vi "Streaming to Asset Example.vi"() -> ()   [LabVIEW 2024]
doc: "Streams multiple channels to a Run."
uses:
  Sift API/Sift Client.lvclass
  Generate Sift Protos/SiftProxy_client/RPC Messages/sift_proxy_v1_ChannelDataType.ctl
  Sift Client.lvlib
  Generate Sift Protos/SiftProxy_client/SiftProxy_client.lvlib
panel:
  out "Running":bool
  out "Flush Error":errorcluster
  in  "Test Channel 2":dbl(slide) scale=0.0..10.0
  in  "Stop":bool
  in  "Test Channel 1":dbl(slide) scale=0.0..10.0
  in  "Test Channel 3":bool
  out "Error":errorcluster
  in  "Organization ID":string
  in  "API Key":string
  in  "API URL":string
  # "Sift Streaming Example"
  # "Instructions\n\n1. Fill in the API URL, API Key, and Organization ID. Visit this URL for more information on authentication\n    https://docs.siftstack.com/docs/api/authentication\n\n\n2. Start the VI\n\n3. Navigate to the Assets page and open the \"LabVIEW-Example\" asset.\n\n4. You should see the test test channels in the run.\n\n5. Click on the Live button and manually adjust the Controls to see the telemetry update.\n\n6. Click Stop to stop the VI."
  # "This example streams data live from LabVIEW.\n\nFill in the information below then open the corresponding Run in Sift\nto see data streaming in Live.\n\nNote: Remembver to hit the \"Live\" button after opening the run."
  # "Adjust these values while streaming"
  # "Hit this to stop the example."
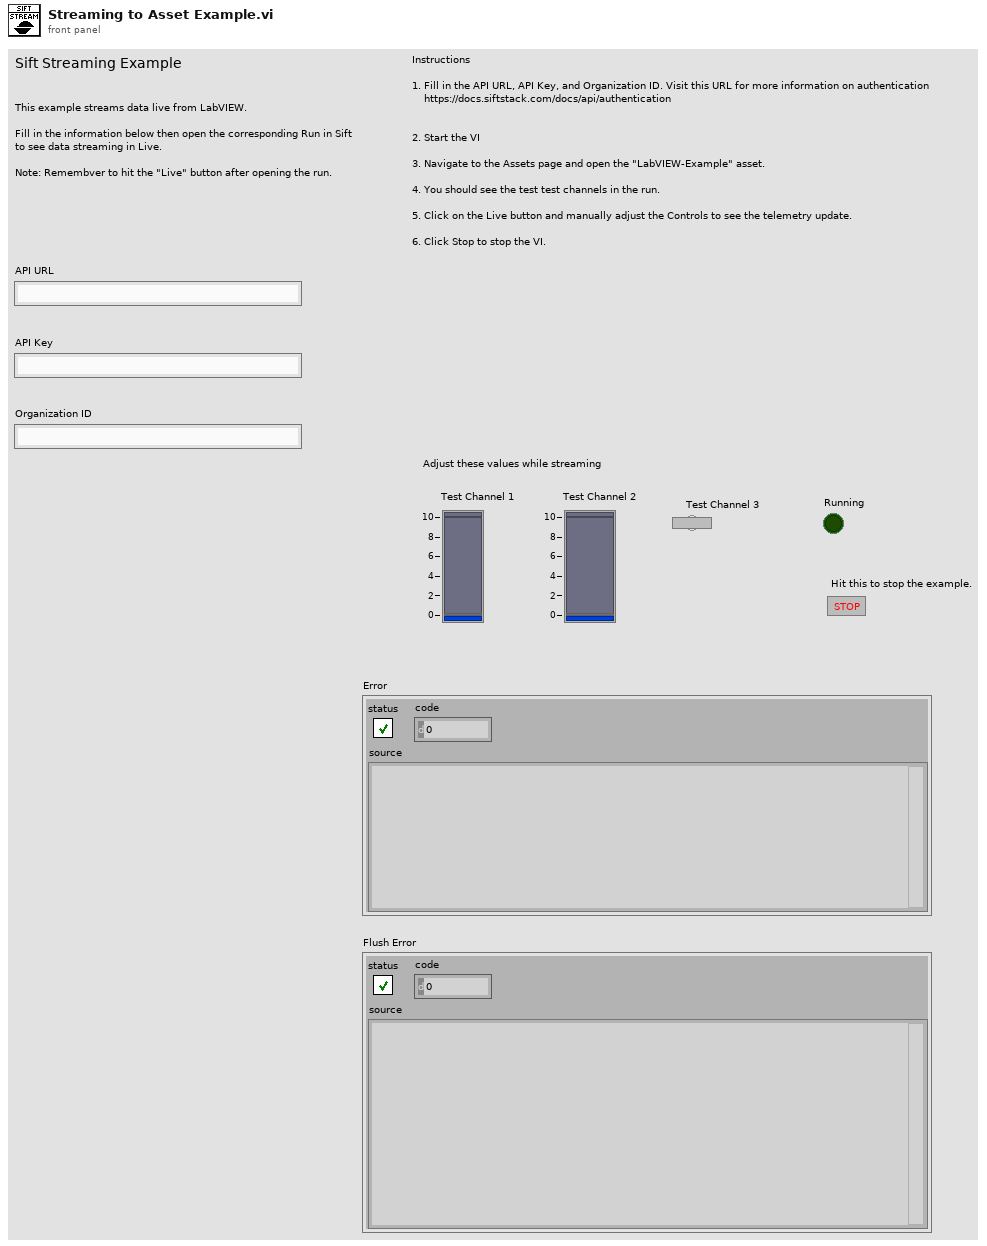
[diagram p1: front panel]
types:
  T1 = typedef "SiftProxy_client.lvlib/sift_proxy_v1_ChannelDataType.ctl" = enum32{"CHANNEL_DATA_TYPE_UNSPECIFIED", "CHANNEL_DATA_TYPE_DOUBLE", "CHANNEL_DATA_TYPE_STRING", "CHANNEL_DATA_TYPE_ENUM", "CHANNEL_DATA_TYPE_BIT_FIELD", "CHANNEL_DATA_TYPE_BOOL", "CHANNEL_DATA_TYPE_FLOAT", "CHANNEL_DATA_TYPE_INT_32", "CHANNEL_DATA_TYPE_UINT_32", "CHANNEL_DATA_TYPE_INT_64", "CHANNEL_DATA_TYPE_UINT_64"}
  T2 = typedef "SiftProxy_client.lvlib/google_protobuf_Timestamp.ctl" = cluster{"seconds":i64, "nanos":i32}
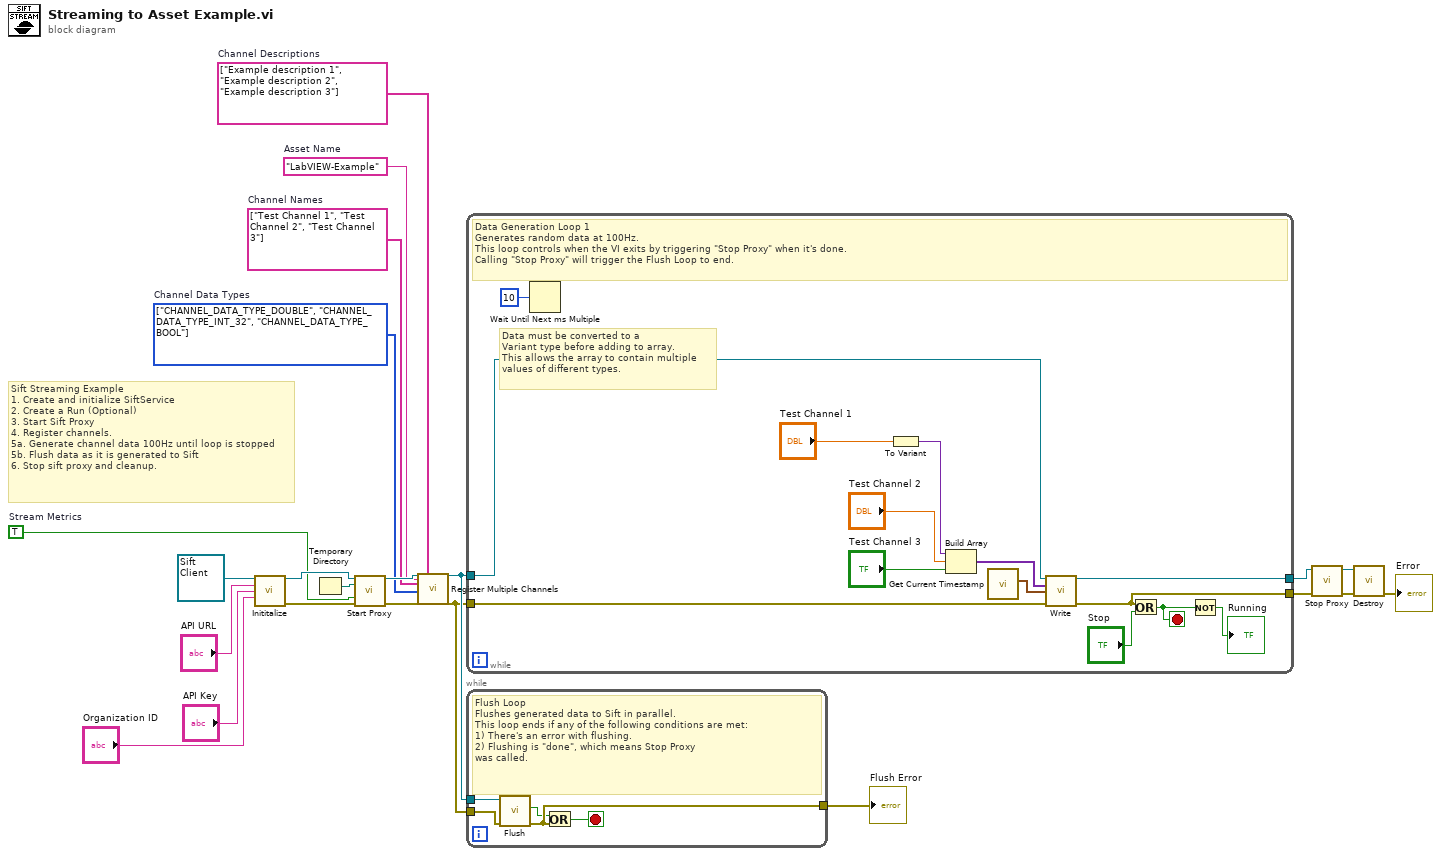
[diagram p0: block diagram]
diagram:
  w7 = "LabVIEW-Example"  # Asset Name
  w9 = T1[] [enum."CHANNEL_DATA_TYPE_DOUBLE", enum."CHANNEL_DATA_TYPE_INT_32", enum."CHANNEL_DATA_TYPE_BOOL"] items=["CHANNEL_DATA_TYPE_UNSPECIFIED", "CHANNEL_DATA_TYPE_DOUBLE", "CHANNEL_DATA_TYPE_STRING", "CHANNEL_DATA_TYPE_ENUM", "CHANNEL_DATA_TYPE_BIT_FIELD", "CHANNEL_DATA_TYPE_BOOL", "CHANNEL_DATA_TYPE_FLOAT", "CHANNEL_DATA_TYPE_INT_32", "CHANNEL_DATA_TYPE_UINT_32", "CHANNEL_DATA_TYPE_INT_64", "CHANNEL_DATA_TYPE_UINT_64"]  # Channel Data Types
  w8 = string[] ["Example description 1", "Example description 2", "Example description 3"]  # Channel Descriptions
  w10 = string[] ["Test Channel 1", "Test Channel 2", "Test Channel 3"]  # Channel Names
  w16 = TRUE  # Stream Metrics
  # "Sift Streaming Example\n1. Create and initialize SiftService\n2. Create a Run (Optional)\n3. Start Sift Proxy\n4. Register channels.\n5a. Generate channel data 100Hz until loop is stopped\n5b. Flush data as it is generated to Sift\n6. Stop sift proxy and cleanup."
  n1 = call-dynamic "Inititalize.vi"("Sift Client in"=refnum<class "Sift Client.lvclass"> refnum ("Sift Client.lvlib:Sift Client.lvclass"), "API URL"="API URL", "API Key"="API Key", "Organization ID"="Organization ID") -> ("Sift Client out"=w18:refnum<class "Sift Client.lvclass">, "error out"=w17:errorcluster)  [unwired: 10 in]
  n2 = Temporary Directory() -> (w1:path)
  n3 = call-dynamic "Start Proxy.vi"("Sift Client in"=w18, "Storage Path"=w1, "Stream Metrics"=w16, "error in (no error)"=w17) -> ("Sift Client out"=w11:refnum<class "Sift Client.lvclass">, "error out"=w12:errorcluster)  [unwired: 10 in]
  n4 = call "Register Multiple Channels.vi"("Sift Client in"=w11, "Asset Name"=w7, "Names"=w10, "Data Types"=w9, "error in (no error)"=w12, "Descriptions"=w8) -> ("Sift Client out"=w4:refnum<class "Sift Client.lvclass">, "error out"=w2:errorcluster)  [unwired: 20 in]
  n5 = while {
    tunnel: w4 -> [w36]
    tunnel: w2 -> [w35]
    tunnel: [w28] -> w6
    tunnel: [w30] -> w5
    stop <- w23 stop-if-true
    # "Data must be converted to a \nVariant type before adding to array.\nThis allows the array to contain multiple \nvalues of different types."
    # "Data Generation Loop 1\nGenerates random data at 100Hz.\nThis loop controls when the VI exits by triggering \"Stop Proxy\" when it's done. \nCalling \"Stop Proxy\" will trigger the Flush Loop to end."
    n6 = Wait Until Next ms Multiple(millisecond multiple=u32 10 ("milliseconds to wait")) -> ()  [unwired: 1 out]
    n7 = To Variant(anything="Test Channel 1") -> (Variant=w33:variant)
    n8 = Build Array(w33, "Test Channel 2", "Test Channel 3") -> (w32:variant[])
    n9 = call "Get Current Timestamp.vi"() -> ("Timestamp"=w31:T2)  [unwired: 11 in]
    n10 = call-dynamic "Write.vi"("Sift Client in"=w36, "Values"=w32, "Timestamp"=w31, "error in (no error)"=w35) -> ("Sift Client out"=w28:refnum<class "Sift Client.lvclass">, "error out"=w30:errorcluster)  [unwired: 10 in]
    n11 = Or(x=w30, y="Stop") -> (x .or. y?=w23:bool)
    n12 = Not(x=w23) -> (.not. x?=→"Running":bool)
  }
  n13 = while {
    tunnel: w4 -> [w41]
    tunnel: [w39] -> w3
    tunnel: w2 -> [w40]
    stop <- w37 stop-if-true
    # "Flush Loop\nFlushes generated data to Sift in parallel.\nThis loop ends if any of the following conditions are met:\n1) There's an error with flushing.\n2) Flushing is \"done\", which means Stop Proxy \nwas called."
    n14 = call-dynamic "Flush.vi"("error in (no error)"=w40, "Sift Client in"=w41) -> ("error out"=w39:errorcluster, "Done"=w38:bool)  [unwired: 7 in, 1 out]
    n15 = Or(x=w38, y=w39) -> (x .or. y?=w37:bool)
  }
  "Flush Error" <- w3
  n16 = call-dynamic "Stop Proxy.vi"("error in (no error)"=w5, "Sift Client in"=w6) -> ("error out"=w15:errorcluster, "Sift Client out"=w14:refnum<class "Sift Client.lvclass">)  [unwired: 7 in, 1 out]
  n17 = call-dynamic "Destroy.vi"("error in (no error)"=w15, "Sift Client in"=w14) -> ("error out"=→"Error":errorcluster)  [unwired: 8 in, 1 out]
